vi "Memory.Pointer.Internal.New.vi"(8 "error in (no error)":errorcluster, 11 "size":u64 format="%08x bytes") -> (0 "error out":errorcluster, 3 "pointer":refnum<class "Memory.Pointer.Internal.lvclass">)   [LabVIEW 2016, in "Memory Manager.lvlib" / "Memory.Pointer.Internal.lvclass"]
doc: "Allocates a new pointer that points to a block of memory that is <b>size</b> bytes in length."
uses:
  Memory.Pointer.Internal.lvclass
  C:/Users/Ryan/Documents/Git/Sourcetree/LabVIEW-Memory-Manager/Source/Library/Classes/Pointer/Memory.Pointer.lvclass
  Pointer/Memory.Pointer.lvclass/Memory.Pointer.ctl
  Pointer/Memory.Pointer.lvclass
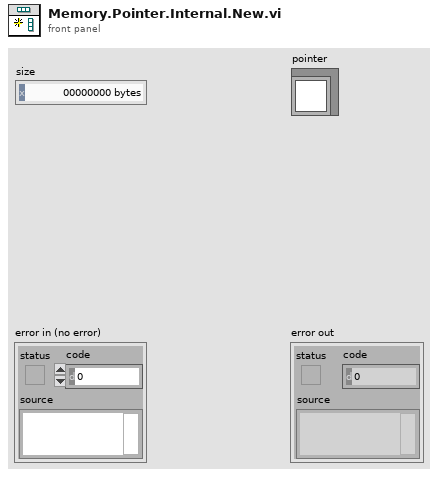
[diagram p1: front panel]
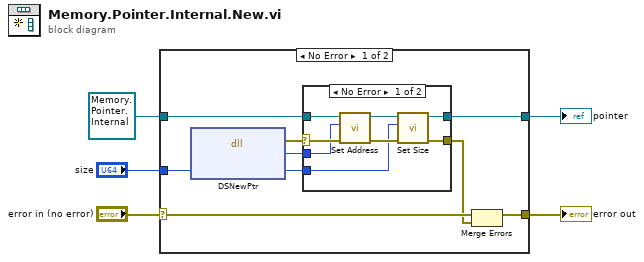
[diagram p0: block diagram]
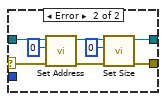
[diagram p2: hidden frame]
diagram:
  n1 = case shown="No Error" "error in (no error)" {
    selector: "error in (no error)" -> [w13 w32]
    tunnel: [w14 w32] -> w5
    tunnel: [w7 w31] -> w4
    tunnel: "size" -> [w8 _]
    tunnel: refnum<class "Memory.Pointer.Internal.lvclass"> refnum ("Pointer") -> [w6 w31]
    frame No Error {
      n2 = dll-call lib="LabVIEW" fn="DSNewPtr"("size"=w8) -> (error out=w10:errorcluster, "pointer"=w12:u64, "size"=w11:u64)  [unwired: 3 in, 1 out]
      n3 = case shown="No Error" w10 {
        selector: w10 -> [w21 w29]
        tunnel: w6 -> [w22 w30]
        tunnel: w12 -> [w20 _]
        tunnel: [w17 w26] -> w7
        tunnel: w11 -> [w15 _]
        tunnel: [w16 w25] -> w9
        frame No Error {
          n4 = call "Set Address.vi"("error in (no error)"=w21, "address"=w20, "Pointer in"=w22) -> ("error out"=w18:errorcluster, "Pointer out"=w19:refnum<class "Memory.Pointer.Internal.lvclass">)  [unwired: 7 in]
          n5 = call "Set Size.vi"("error in (no error)"=w18, "size"=w15, "Pointer in"=w19) -> ("error out"=w16:errorcluster, "Pointer out"=w17:refnum<class "Memory.Pointer.Internal.lvclass">)  [unwired: 7 in]
        }
        frame Error {
          n6 = call "Set Address.vi"("error in (no error)"=w29, "address"=u64 0, "Pointer in"=w30) -> ("error out"=w27:errorcluster, "Pointer out"=w28:refnum<class "Memory.Pointer.Internal.lvclass">)  [unwired: 7 in]
          n7 = call "Set Size.vi"("error in (no error)"=w27, "size"=u64 0, "Pointer in"=w28) -> ("error out"=w25:errorcluster, "Pointer out"=w26:refnum<class "Memory.Pointer.Internal.lvclass">)  [unwired: 7 in]
        }
      }
      n8 = Merge Errors(w13, w9) -> (w14:errorcluster)
    }
    frame Error {
    }
  }
  "error out" <- w5
  "pointer" <- w4
